vi "Write Event.vi"(8 "error in (no error)":errorcluster, 10 "Event":cluster{"Stop":refnum<user-event>}, 11 "Execute":refnum<class "Execute.lvclass">) -> (0 "error out":errorcluster, 3 "Execute":refnum<class "Execute.lvclass">)   [LabVIEW 2018, in "QMH_Class.lvlib" / "TestManager.lvlib" / "Execute.lvclass"]
uses:
  Execute.lvclass
  Execute.lvclass/Execute.ctl
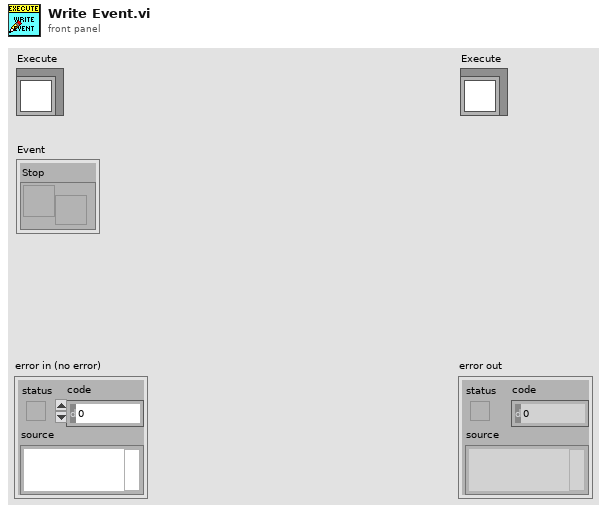
[diagram p1: front panel]
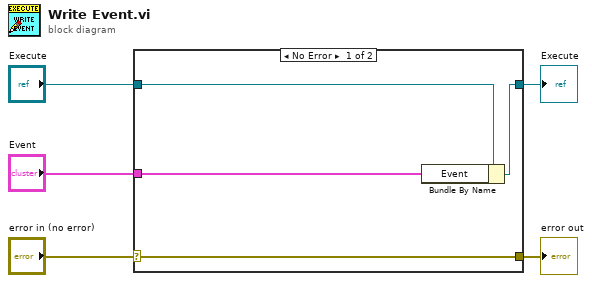
[diagram p0: block diagram]
diagram:
  n1 = case shown="No Error" "error in (no error)" {
    selector: "error in (no error)" -> [w9 w10]
    tunnel: [w9 w10] -> w4
    tunnel: [w7 w11] -> w2
    tunnel: "Execute" -> [w8 w11]
    tunnel: "Event" -> [w6 _]
    frame No Error {
      n2 = Bundle By Name(cluster=w8, "Event"=w6) -> (w7:refnum<class "Execute.lvclass">)
    }
    frame Error {
    }
  }
  "error out" <- w4
  "Execute" <- w2
